vi "GetMessageRef.vi"(8 "error in":errorcluster, 11 "error processor in":refnum<class "ErrorProcessor.lvclass">) -> (0 "error out":errorcluster, 2 "message ref":refnum<class "CLM_PriorityLocalMessage.lvclass">, 3 "error processor out":refnum<class "ErrorProcessor.lvclass">)   [LabVIEW 2013, in "CLM_ErrorHandler.lvlib" / "ErrorProcessor.lvclass"]
uses:
  ErrorProcessor.lvclass
  <vilib>/CLM/LocalMessenger/PriorityLocalMessage/CLM_PriorityLocalMessage.lvclass
  ErrorProcessor.lvclass/ErrorProcessor.ctl
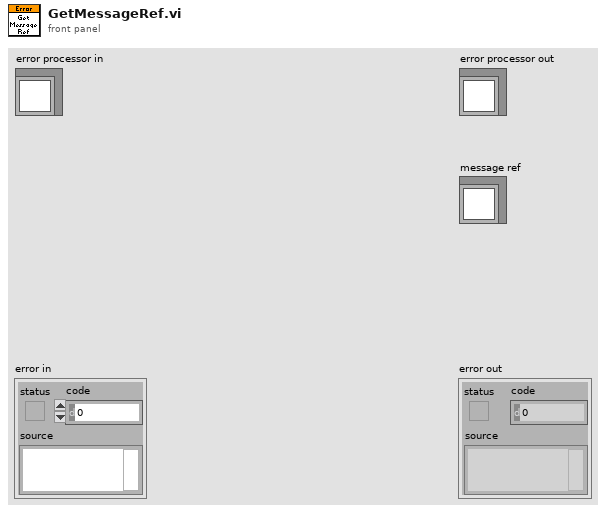
[diagram p1: front panel]
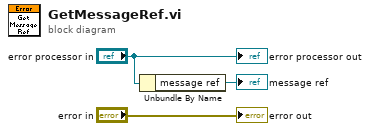
[diagram p0: block diagram]
diagram:
  n1 = Unbundle By Name("error processor in") -> ("message ref"=→"message ref":refnum<class "CLM_PriorityLocalMessage.lvclass">)
  "error out" <- "error in"
  "error processor out" <- "error processor in"
